vi "Compound Destroy.vi"(8 "error in (no error)":errorcluster, 11 "Compound DVR in":refnum<data-value>) -> (0 "error out":errorcluster)   [LabVIEW 2012, in "MDSplus.lvlib"]
uses:
  <vilib>/MDSplus/Library/MDSplus.lvlib
  <vilib>/MDSplus/Classes/Data_Class/Compound_Class/Compound.lvclass
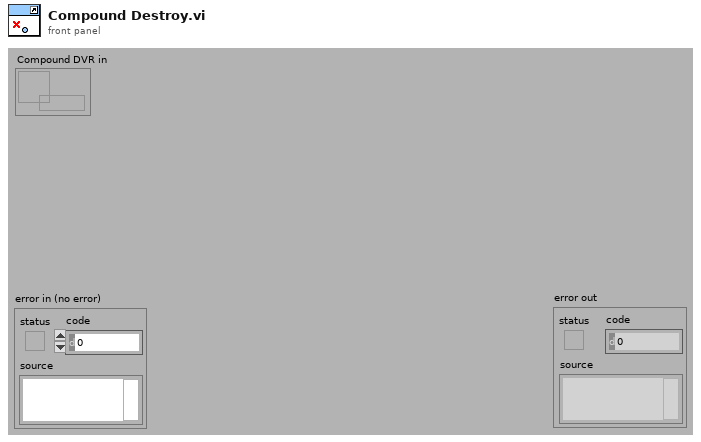
[diagram p1: front panel]
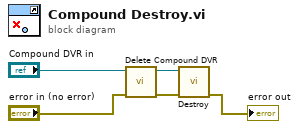
[diagram p0: block diagram]
diagram:
  n1 = call <vilib>:"Delete Compound DVR.vi"("error in (no error)"="error in (no error)", "Compound DVR in"="Compound DVR in") -> ("error out"=w2:errorcluster, "Compound out"=w3:refnum<class "Compound.lvclass">)  [unwired: 8 in]
  n2 = call-dynamic "Destroy.vi"("error in (no error)"=w2, "Compound in"=w3) -> ("error out"=→"error out":errorcluster)  [unwired: 9 in]
